vi "parseMsgBatteryState.vi"(8 "error in":errorcluster, 11 "msg":string) -> (0 "error out":errorcluster, 3 "batteryState":T1)   [LabVIEW 2018]
uses:
  <userlib>/ROS for LabVIEW Software/ROS/MessageParsing/std_msgs/subs/parse_float32_scalar.vi
  <userlib>/ROS for LabVIEW Software/ROS/MessageParsing/std_msgs/subs/parse_u8_scalar.vi
  <userlib>/ROS for LabVIEW Software/ROS/MessageParsing/std_msgs/subs/parse_bool_scalar.vi
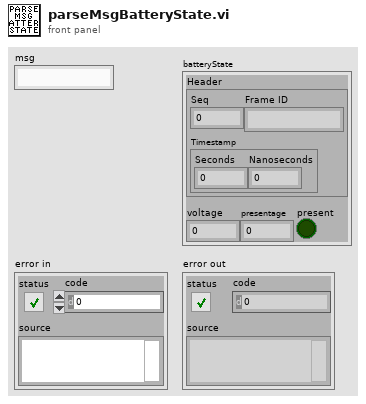
[diagram p1: front panel]
types:
  T1 = cluster{"Header":cluster{"Seq":u32, "Frame ID":string, "Timestamp":cluster{"Seconds":i32, "Nanoseconds":i32}}, "voltage":sgl, "presentage":sgl, "present":bool}
  T2 = cluster{"Seq":u32, "Frame ID":string, "Timestamp":cluster{"Seconds":i32, "Nanoseconds":i32}}
  T3 = cluster{"Header":cluster{"Seq":u32, "Frame ID":string, "Timestamp":cluster{"Seconds":i32, "Nanoseconds":i32}}, "number":sgl, "number":sgl, "bool":bool}
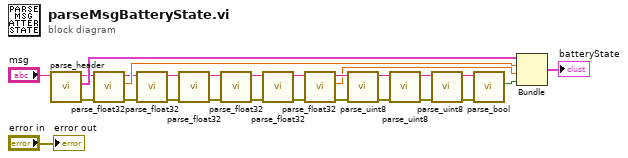
[diagram p0: block diagram]
diagram:
  n1 = call <userlib>:"parse_header.vi"("msg in"="msg") -> ("error out"=w16:errorcluster, "Header"=w9:T2, "msg out"=w3:string)  [unwired: 4 in]
  n2 = call-poly <userlib>:"parse_float32.vi"("error in"=w16, "msg in"=w3) -> ("error out"=w17:errorcluster, "number"=w10:sgl, "msg out"=w4:string)  [unwired: 3 in]
  n3 = call-poly <userlib>:"parse_float32.vi"("error in"=w17, "msg in"=w4) -> ("error out"=w18:errorcluster, "msg out"=w5:string)  [unwired: 3 in, 1 out]
  n4 = call-poly <userlib>:"parse_float32.vi"("error in"=w18, "msg in"=w5) -> ("error out"=w19:errorcluster, "msg out"=w8:string)  [unwired: 3 in, 1 out]
  n5 = call-poly <userlib>:"parse_float32.vi"("error in"=w19, "msg in"=w8) -> ("error out"=w20:errorcluster, "msg out"=w7:string)  [unwired: 3 in, 1 out]
  n6 = call-poly <userlib>:"parse_float32.vi"("error in"=w20, "msg in"=w7) -> ("error out"=w21:errorcluster, "msg out"=w6:string)  [unwired: 3 in, 1 out]
  n7 = call-poly <userlib>:"parse_float32.vi"("error in"=w21, "msg in"=w6) -> ("error out"=w22:errorcluster, "number"=w11:sgl, "msg out"=w13:string)  [unwired: 3 in]
  n8 = call-poly <userlib>:"parse_uint8.vi"("error in"=w22, "msg in"=w13) -> ("error out"=w23:errorcluster, "msg out"=w14:string)  [unwired: 3 in, 1 out]
  n9 = call-poly <userlib>:"parse_uint8.vi"("error in"=w23, "msg in"=w14) -> ("error out"=w24:errorcluster, "msg out"=w15:string)  [unwired: 3 in, 1 out]
  n10 = call-poly <userlib>:"parse_uint8.vi"("error in"=w24, "msg in"=w15) -> ("error out"=w26:errorcluster, "msg out"=w25:string)  [unwired: 3 in, 1 out]
  n11 = call-poly <userlib>:"parse_bool.vi"("error in"=w26, "msg in"=w25) -> ("bool"=w27:bool)  [unwired: 3 in, 2 out]
  n12 = Bundle("Header"=w9, "number"=w10, "number"=w11, "bool"=w27) -> (→"batteryState":T3)  [unwired: 1 in]
  "error out" <- "error in"
